vi "loop.vi"() -> ()   [LabVIEW 2017]
uses:
  <vilib>/FPGAPlugInAG/myRIO-1900/niLvFpga_Open_myRIO-1900.vi
  <vilib>/rvi/interface/common/dynamic/niFpgaDynamicAddResources.vi
  <vilib>/Utility/error.llb/Error Cluster From Error Code.vi
  <vilib>/rvi/errors/niLvFpgaAdjustHostInterfaceError.vi
  <vilib>/FPGAPlugInAG/Dynamic/niLvFpga_Close_Dynamic.vi
  <vilib>/rvi/interface/nirviOpenFPGA/nirviOpenFPGA.xnode
  FPGA Bitfiles/test-3-vehicleco_FPGATarget_Fpgatest3_-vhTzbdOOx4.lvbitx
  FPGA_controller.vi
  <vilib>/rvi/interface/nirviReadWriteControl/nirviReadWriteControl.xnode
  <vilib>/rvi/interface/nirviCloseFPGA/nirviCloseFPGA.xnode
  NiFpgaLv.dll
  <vilib>/rvi/interface/Simulation/niFpgaSimulationCallBeginRW.vi
panel:
  out "Iteration":i32
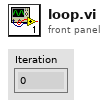
[diagram p1: front panel]
types:
  T1 = cluster{"Boolean array[0]":bool, "Boolean array[1]":bool, "Boolean array[2]":bool, "Boolean array[3]":bool, "Boolean array[4]":bool, "Boolean array[5]":bool}
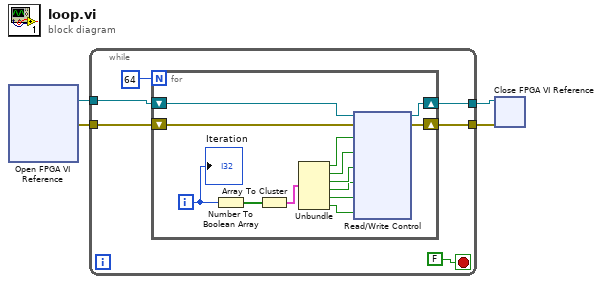
[diagram p0: block diagram]
diagram:
  n1 = xnode "Open FPGA VI Reference"() -> ("FPGA VI Reference Out"=w4:refnum<k20>, "error out"=w3:errorcluster)  [unwired: 2 in]
  n2 = while {
    tunnel: w4 -> [w8]
    tunnel: w3 -> [w7]
    tunnel: [w6] -> w2
    tunnel: [w5] -> w1
    stop <- FALSE stop-if-true
    n3 = for {
      N: 64 -> [_]
      shift-right: [w17] -> w5
      shift-left: w7 -> [w19]
      shift-right: [w18] -> w6
      shift-left: w8 -> [w20]
      i -> [w21]
      n4 = Number To Boolean Array(number=w21) -> (Boolean array=w23:bool[])
      n5 = Array To Cluster(array=w23) -> (cluster=w22:T1)
      n6 = Unbundle(w22) -> ("Boolean array[0]"=w16:bool, "Boolean array[1]"=w15:bool, "Boolean array[2]"=w14:bool, "Boolean array[3]"=w13:bool, "Boolean array[4]"=w12:bool, "Boolean array[5]"=w11:bool)
      n7 = xnode "Read/Write Control"("FPGA VI Reference In"=w20, "error in"=w19, "Input_1"=w16, "Input_2"=w15, "Input_3"=w14, "Input_4"=w13, "Input_5"=w12, "Input_6"=w11) -> ("FPGA VI Reference Out"=w18:refnum<k20>, "error out"=w17:errorcluster)
      "Iteration" <- w21
    }
  }
  n8 = xnode "Close FPGA VI Reference"("FPGA VI Reference In"=w2, "error in"=w1) -> ()  [unwired: 1 out]
